vi "Close.vi"(8 "error in (no error)":errorcluster, 11 "dbcDotNet in":refnum<class "ORM_DBC_dotNet.lvclass">) -> (0 "error out":errorcluster)   [LabVIEW 2020, in "ORM_DBC_dotNet.lvlib" / "ORM_DBC_dotNet.lvclass"]
uses:
  ORM_DBC_dotNet.lvclass
  ORM_DBC_dotNet.lvclass/ORM_DBC_dotNet.ctl
  Read connection.vi
  Read transactions.vi
  System.Data
  <vilib>/Viviota/shared/ORM.lvlibp/ORM/DbConnection/DbConnection.lvclass
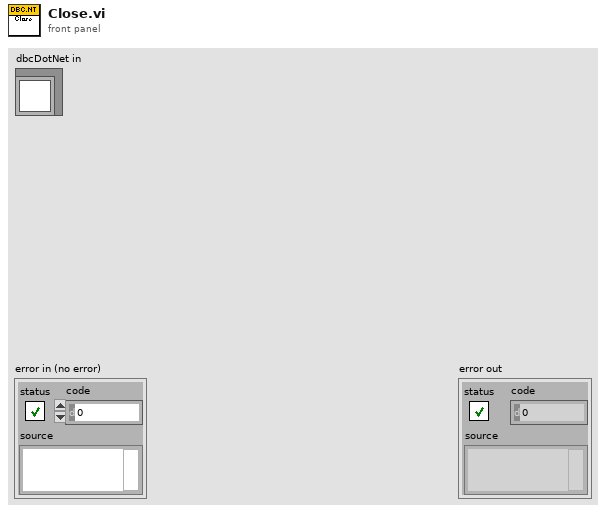
[diagram p1: front panel]
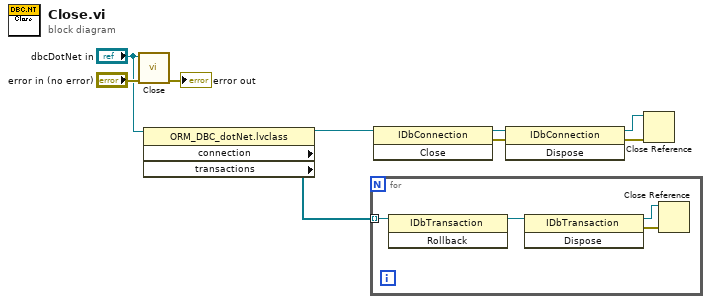
[diagram p0: block diagram]
diagram:
  n1 = call-parent "Close.vi"("error in (no error)"="error in (no error)", "DbConnection in"="dbcDotNet in") -> ("error out"=→"error out":errorcluster)  [unwired: 9 in]
  n2 = property class="ORM_DBC_dotNet.lvclass"(reference="dbcDotNet in") -> ("connection"=w3:refnum<k24>, "transactions"=w1:refnum<k24>[])  [unwired: 1 in, 2 out]
  n3 = for {
    tunnel: w1 -> [w10] mode=indexing
    n4 = invoke class="IDbTransaction" method="Rollback"(reference=w10) -> (reference out=w13:refnum<k24>)  [unwired: 2 in, 2 out]
    n5 = invoke class="IDbTransaction" method="Dispose"(reference=w13) -> (reference out=w11:refnum<k24>, error out=w12:errorcluster)  [unwired: 2 in, 1 out]
    n6 = Close Reference(reference=w11, error in (no error)=w12) -> ()  [unwired: 1 out]
  }
  n7 = invoke class="IDbConnection" method="Close"(reference=w3) -> (reference out=w7:refnum<k24>, error out=w4:errorcluster)  [unwired: 2 in, 1 out]
  n8 = invoke class="IDbConnection" method="Dispose"(reference=w7, error in=w4) -> (reference out=w5:refnum<k24>, error out=w6:errorcluster)  [unwired: 1 in, 1 out]
  n9 = Close Reference(reference=w5, error in (no error)=w6) -> ()  [unwired: 1 out]
